vi "Group ID to Tree Items.vi"(8 "error in (no error)":errorcluster, 9 "Group ID":string, 11 "Application Data in":T2) -> (0 "error out":errorcluster, 1 "Settings":T1, 2 "Item":T1, 3 "Application Data out":T2)   [LabVIEW 2017, in "DSF Data Viewer.lvlib"]
uses:
  DSF Data Viewer.lvlib
  Tree Item Type.ctl
  Core/DSF Configuration API/Configuration Session.lvclass
  Core/DSF Configuration API/Public/Read Item/Read Group.vi
  Core/DSF Configuration API/Public/Read Item/Read Settings.vi
  Main VI/Application Data.ctl
  Tree Item.ctl
  Main VI/View Mode.ctl
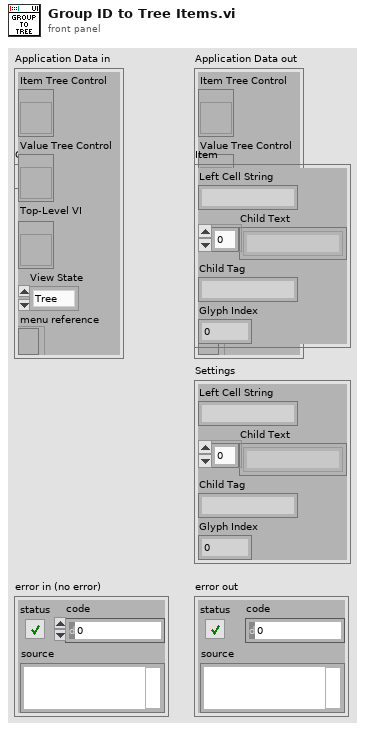
[diagram p1: front panel]
types:
  T1 = typedef "DSF Data Viewer.lvlib/Tree Item.ctl" = cluster{"Left Cell String":string, "Child Text":string[], "Child Tag":string, "Glyph Index":i32}
  T2 = typedef "DSF Data Viewer.lvlib/Application Data.ctl" = cluster{"Item Tree Control":refnum<vi>, "Value Tree Control":refnum<vi>, "Top-Level VI":refnum<vi>, "View State":T3, "menu reference":refnum<k9>}
  T3 = typedef "DSF Data Viewer.lvlib/View Mode.ctl" = enum16{"Tree", "List"}
  T4 = typedef "DSF Data Viewer.lvlib/Tree Item Type.ctl" = enum16{"Plugin", "Group", "Transfer", "Channel", "Setting"}
  T5 = typedef "DSF Core.lvlib/DSF Group Info.ctl" = cluster{"direction":T6, "timing":T7, "transfer ids":string[], "settings id":string, "thread":i32}
  T6 = typedef "DSF Core.lvlib/DSF Direction.ctl" = enum8{"Tx", "Rx"}
  T7 = typedef "DSF Core.lvlib/DSF Timing Info.ctl" = cluster{"priority":u64, "decimation":u64, "offset":u64}
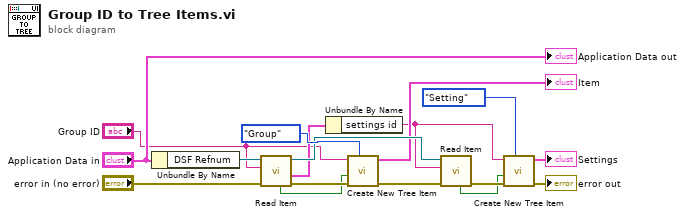
[diagram p0: block diagram]
diagram:
  n1 = Unbundle By Name("Application Data in") -> ("DSF Refnum"=w7:refnum<class "Configuration Session.lvclass">)
  n2 = call-poly "Read Item.vi"("error in (no error)"="error in (no error)", "Group ID"="Group ID", "Configuration Session in"=w7) -> ("error out"=w13:errorcluster, "value"=w10:T5, "Configuration Session out"=w12:refnum<class "Configuration Session.lvclass">, "found?"=w2:bool)  [unwired: 5 in]
  n3 = Unbundle By Name(w10) -> ("settings id"=w3:string)
  n4 = call "Create New Tree Item.vi"("Item Type"=Tree_Item_Type."Group", "error in"=w13, "found?"=w2, "Left Cell String"="Group ID") -> ("error out"=w14:errorcluster, "Item"=→"Item":T1)  [unwired: 6 in]
  n5 = call-poly "Read Item.vi"("error in (no error)"=w14, "Settings ID"=w3, "Configuration Session in"=w12) -> ("error out"=w15:errorcluster, "found?"=w1:bool)  [unwired: 5 in, 2 out]
  n6 = call "Create New Tree Item.vi"("Item Type"=Tree_Item_Type."Setting", "error in"=w15, "found?"=w1, "Left Cell String"=w3) -> ("error out"=→"error out":errorcluster, "Item"=→"Settings":T1)  [unwired: 6 in]
  "Application Data out" <- "Application Data in"
